vi "MultiBalloon Controller.vi"() -> ()   [LabVIEW 2018]
uses:
  CollectionSupport.lvlib
panel:
  in  "Balloon 2":bool
  in  "Balloon 1":bool
  in  "Delay":u32 max=1000 step=50
  out "Stopped?":bool
  out "Waveform Chart":dynamicdata(graph)
  in  "Stop Button":bool
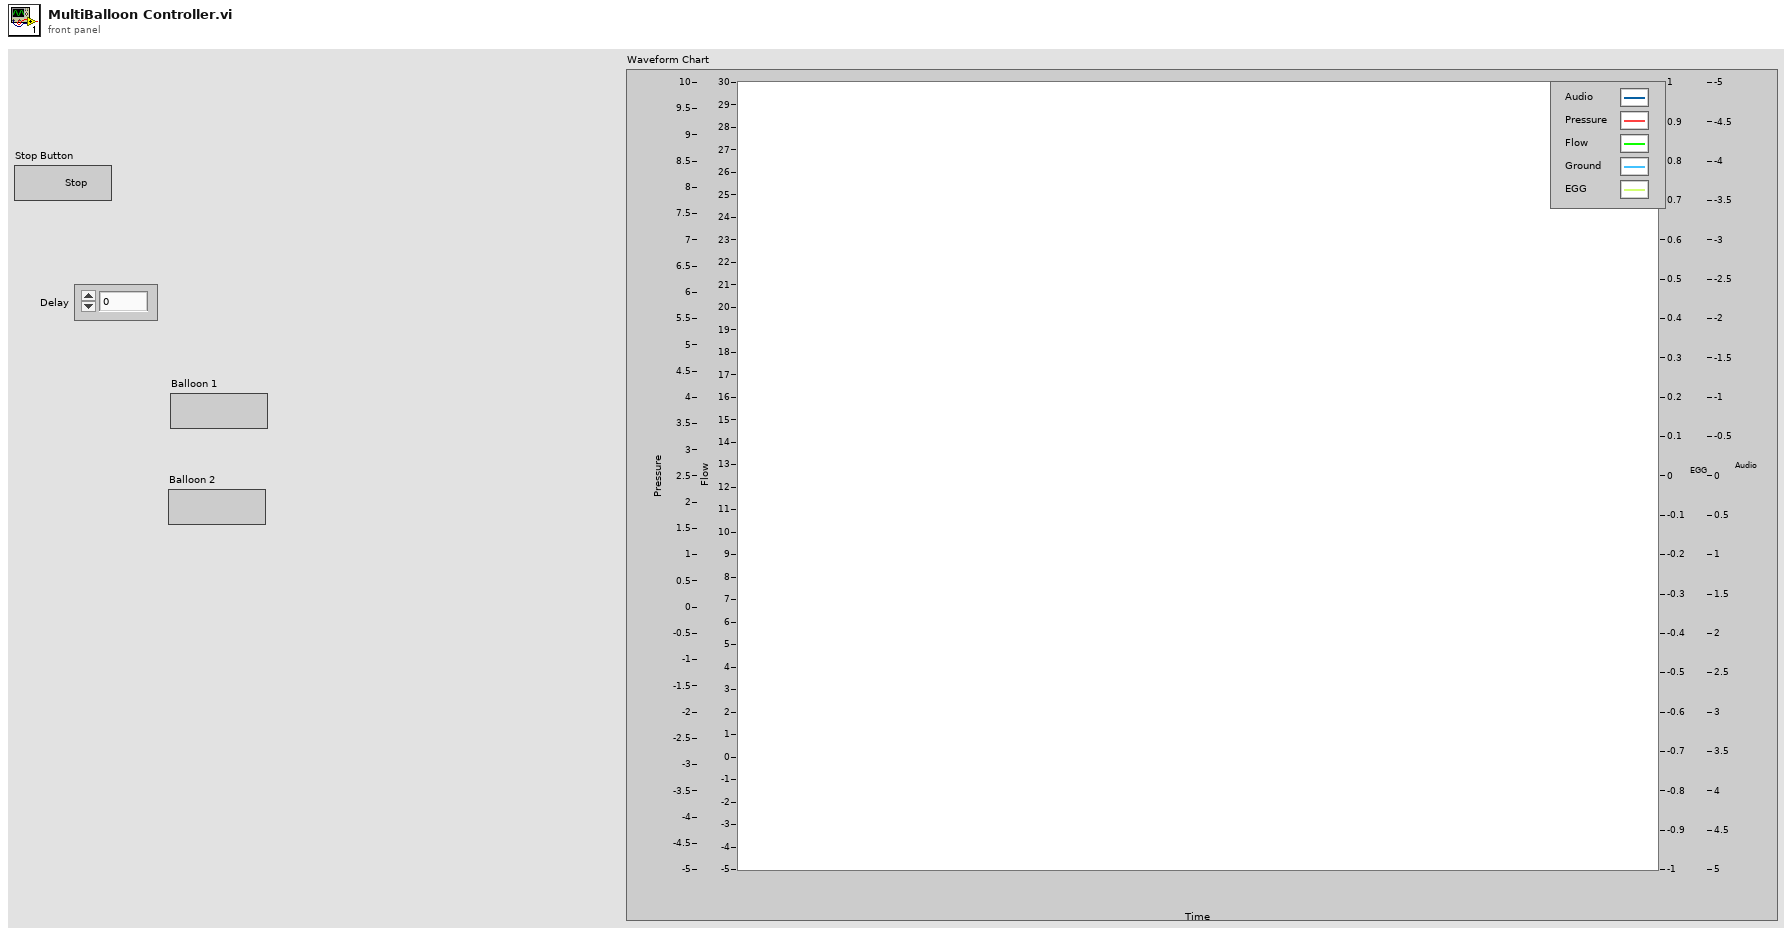
[diagram p1: front panel]
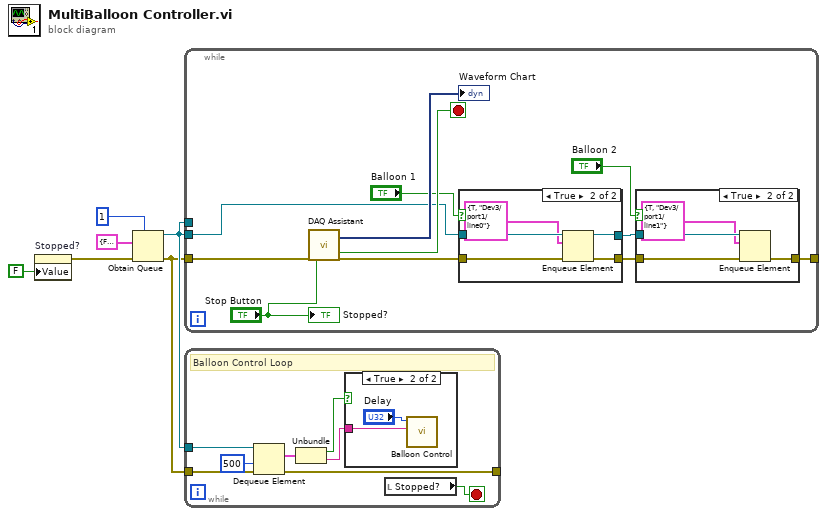
[diagram p0: block diagram]
diagram:
  n1 = property on="Stopped?" class="Bool (strict)"("Value"=FALSE ("Stopped?")) -> (error out=w1:errorcluster)  [unwired: 2 in, 1 out]
  n2 = Obtain Queue(max queue size (-1, unlimited)=1, element data type=cluster{bool, "lines":tag} {FALSE, "lines"="Dev3/port1/line0"}, error in (no error)=w1) -> (queue out=w5:refnum<queue>, error out=w2:errorcluster)  [unwired: 2 in, 1 out]
  n3 = while {
    tunnel: w5 -> [_]
    tunnel: w5 -> [w14]
    tunnel: [w11] -> _
    tunnel: w2 -> [w8]
    stop <- w17 stop-if-true
    n4 = call "DAQ Assistant"("error in"=w8, "stop (F)"="Stop Button") -> ("data"=→"Waveform Chart":dynamicdata, "stopped"=w17:bool, "error out"=w13:errorcluster)  [unwired: 14 in, 1 out]
    n5 = case shown="True" "Balloon 1" {
      tunnel: w14 -> [w23 w29]
      tunnel: w13 -> [w24 w27]
      tunnel: [w24 w26] -> w12
      tunnel: [w23 w25] -> w7
      frame False {
      }
      frame True {
        n6 = Enqueue Element(queue=w29, element=cluster{bool, "lines":tag} {TRUE, "lines"="Dev3/port1/line0"}, error in (no error)=w27) -> (queue out=w25:refnum<queue>, error out=w26:errorcluster)  [unwired: 1 in, 1 out]
      }
    }
    n7 = case shown="True" "Balloon 2" {
      tunnel: w7 -> [_ w22]
      tunnel: w12 -> [w18 w20]
      tunnel: [w18 w19] -> w11
      frame False {
      }
      frame True {
        n8 = Enqueue Element(queue=w22, element=cluster{bool, "lines":tag} {TRUE, "lines"="Dev3/port1/line1"}, error in (no error)=w20) -> (error out=w19:errorcluster)  [unwired: 1 in, 2 out]
      }
    }
    "Stopped?" <- "Stop Button"
  }
  n9 = while {
    tunnel: [w37] -> _
    tunnel: w2 -> [w36]
    tunnel: w5 -> [w34]
    stop <- w35 stop-if-true
    # "Balloon Control Loop"
    n10 = Dequeue Element(queue=w34, timeout in ms (-1)=500, error in (no error)=w36) -> (element=w33:cluster{bool, "lines":tag}, error out=w37:errorcluster)  [unwired: 2 out]
    n11 = Unbundle(w33) -> (w32:bool, "lines"=w31:tag)
    n12 = case shown="True" w32 {
      tunnel: w31 -> [_ w38]
      frame False {
      }
      frame True {
        n13 = call "Balloon Control.vi"("lines"=w38, "Delay (ms)"="Delay") -> ()  [unwired: 10 in]
      }
    }
    n14 = local read "Stopped?"() -> (w35:bool)
  }
